vi "Read Ethernet Configuration.vi"(8 "error in (no error)":errorcluster, 11 "VGC in":refnum<class "PL Inficon VGC.lvclass">) -> (0 "error out":errorcluster, 1 "ip address":string, 2 "dhcp":u32(ring) items=["disabled", "enabled"], 3 "VGC out":refnum<class "PL Inficon VGC.lvclass">, 4 "default gateway":string, 5 "subnet mask":string)   [LabVIEW 2015, in "PL Inficon VGC.lvclass"]
doc: "Reads Ethernet configuration."
uses:
  PL Inficon VGC.lvclass
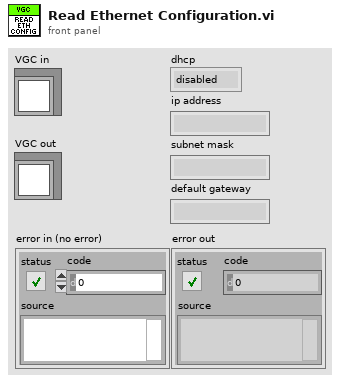
[diagram p1: front panel]
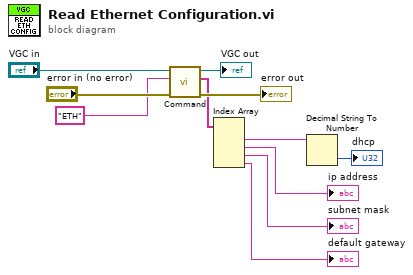
[diagram p0: block diagram]
diagram:
  n1 = call "Command.vi"("error in (no error)"="error in (no error)", "command"="ETH" ("format string"), "VGC in"="VGC in") -> ("error out"=→"error out":errorcluster, "response data"=w5:string[], "VGC out"=→"VGC out":refnum<class "PL Inficon VGC.lvclass">)  [unwired: 6 in]
  n2 = Index Array(array=w5) -> (element #1=w6:string, element #2=→"ip address":string, element #3=→"subnet mask":string, element #4=→"default gateway":string)  [unwired: 4 in]
  n3 = Decimal String To Number(string=w6) -> (number=→"dhcp":i32)  [unwired: 2 in, 1 out]
